vi "Add stage type info.vi"(9 "Stage types in":string[][](array[string]), 10 "Data in":T2(array[cluster]), 11 "Drive letters in":string[](array[string])) -> (3 "Array out":T2(array[cluster]))   [LabVIEW 2019]
uses:
  Class/Controller/Serial parameters.ctl
  Class/Controller/Controller.lvclass
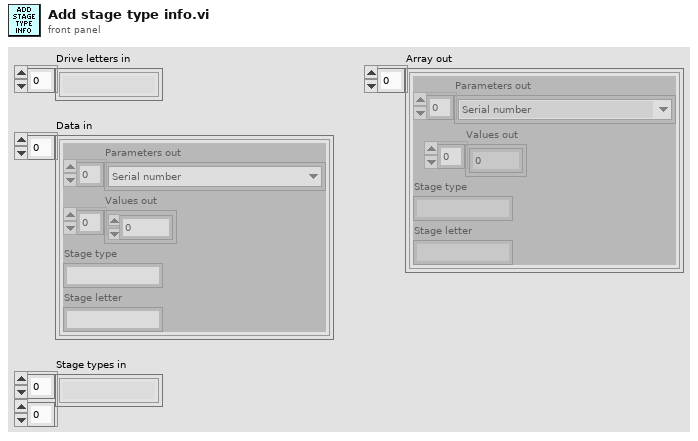
[diagram p1: front panel]
types:
  T1 = typedef "Controller.lvclass/Serial parameters.ctl" = enum16{"Serial number", "Software number", "Type of stage", "Status", "Frequency", "Encoder position", "Desired position", "Info", "Phase correction", "Timestamp", "Proportional control factor", "Sync", "XRT1", "XRT3", "XRTA", "XLS1", "XLS3", "XLA1", "XLA3"}
  T2 = cluster{"Parameters out":T1[], "Values out":i32[], "Stage type":string, "Stage letter":string}[]
  T3 = cluster{"Parameters out":T1[], "Values out":i32[], "Stage type":string, "Stage letter":string}
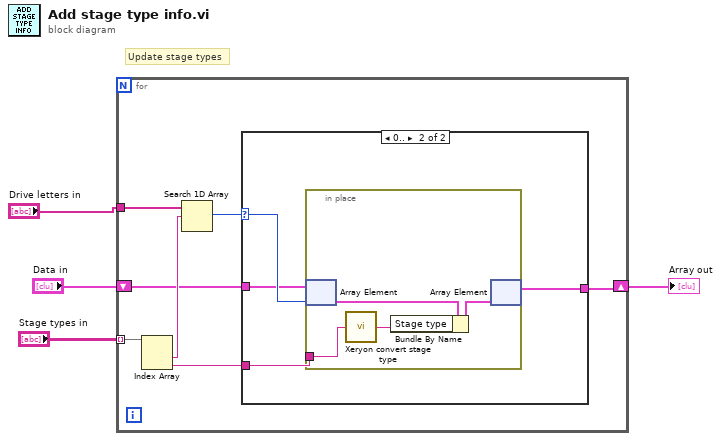
[diagram p0: block diagram]
diagram:
  # "Update stage types"
  n1 = for {
    shift-right: [w5] -> w4
    shift-left: "Data in" -> [w7]
    tunnel: "Stage types in" -> [w11] mode=indexing
    tunnel: "Drive letters in" -> [w10]
    n2 = Index Array(array=w11) -> (element #1=w9:string, element #2=w6:string)  [unwired: 2 in]
    n3 = Search 1D Array(1D array=w10, element=w9) -> (index of element=w8:i32)  [unwired: 1 in]
    n4 = case shown="0.." w8 {
      selector: w8 -> [_ w16]
      tunnel: w7 -> [w12 w15]
      tunnel: w6 -> [_ w14]
      tunnel: [w12 w13] -> w5
      frame -1, Default {
      }
      frame 0.. {
        n5 = in-place {
          in-place-border: w14 -> [w18]
          n6 = in-place-array #1(w15, w16) -> (w20:T3)
          n7 = call "Xeryon convert stage type.vi"("Stage type in"=w18) -> ("Stage type out"=w17:string)  [unwired: 4 in]
          n8 = Bundle By Name(cluster=w20, "Stage type"=w17) -> (w19:T3)
          n9 = in-place-array #1(w19) -> (w13:T2)  [unwired: 1 out]
        }
      }
    }
  }
  "Array out" <- w4
